vi "LHF.DB.Mongo.Util.VariantToQuery.vi"(0 "Equal":variant, 5 "error in (no error)":errorcluster) -> (14 ".NET Refnum out":refnum<k24>, 19 "error out":errorcluster)   [LabVIEW 2013, in "LHF.DB.Mongo.lvclass"]
uses:
  LHF.DB.Mongo.lvclass
  C:/Users/Ricardo/Desktop/Projetos/LabVIEW-MongoDB/src/Driver/MongoDB.Driver.dll
  LabVIEW-MongoDB/src/Driver/MongoDB.Driver.dll
  C:/Users/Ricardo/Desktop/Projetos/LabVIEW-MongoDB/src/Driver/MongoDB.Bson.dll
  LabVIEW-MongoDB/src/Driver/MongoDB.Bson.dll
  <userlib>/_OpenG.lib/string/string.llb/Trim Whitespace (String)__ogtk.vi
  <vilib>/Utility/VariantDataType/VariantType.lvlib
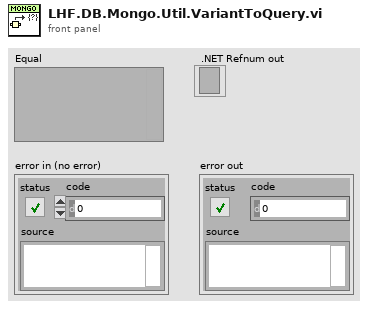
[diagram p1: front panel]
types:
  T1 = typedef "VariantType.lvlib/Type.ctl" = enum8{"Invalid Type", "Void", "I8", "I16", "I32", "I64", "U8", "U16", "U32", "U64", "Single Float", "Double Float", "Extended Float", "Single Complex", "Double Complex", "Extended Complex", "Enum U8", "Enum U16", "Enum U32", "Enum U64", "Single Float With Unit", "Double Float With Unit", "Extended Float With Unit", "Single Complex with Unit", "Double Complex with Unit", "Extended Complex with Unit", "Boolean", "String", "Path", "Picture", "Tag", "Array", "Cluster", "Variant", "LV Variant", "Waveform", "Timestamp", "Digital Waveform", "Digital Data", "ExpressData", "Refnum", "External Data", "VI", "Poly VI", "LabVIEW Class Instance", "Fixed Point"}
  T2 = enum16{"$eq:", "$ne:", "$lte:", "$lt", "$gte:", "$gt:", "<=", "<", ">=", ">", "!=", "==", "!*", "*"}
  T3 = enum16{"$and:", "$and", "&&", "$or:", "$or", "||"}
  T4 = typedef "LHF.DB.Mongo.lvclass/LHF.DB.Mongo.Typedef.VariantData.ctl" = cluster{"Type Enum":T1, "Name":string, "Variant":variant}
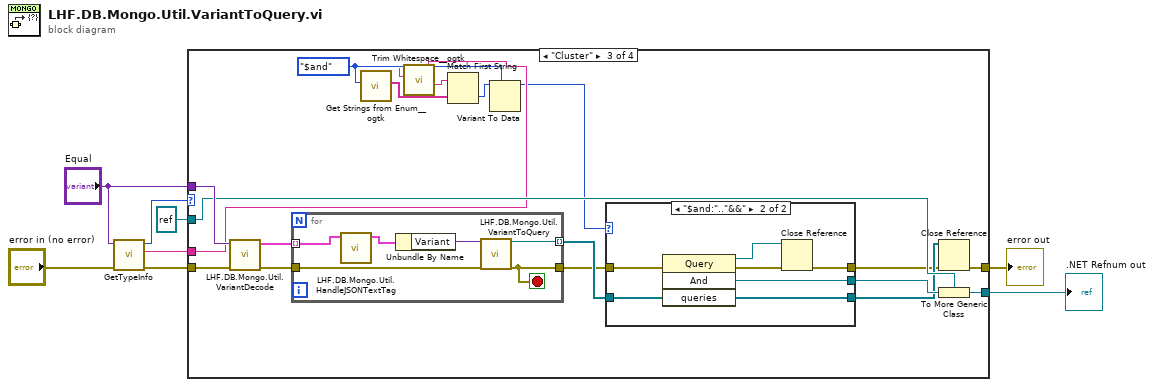
[diagram p0: block diagram]
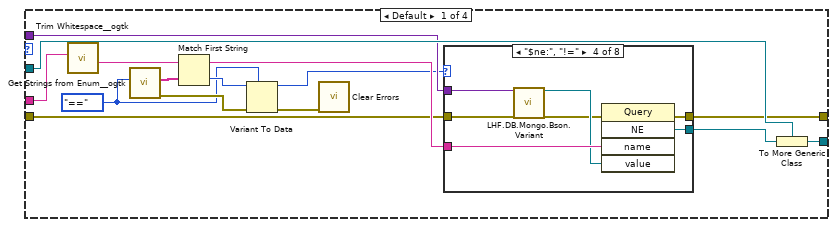
[diagram p2: hidden frame]
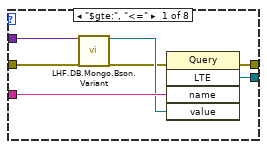
[diagram p3: hidden frame]
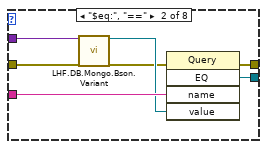
[diagram p4: hidden frame]
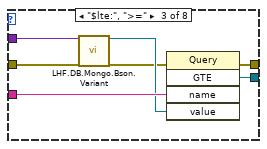
[diagram p5: hidden frame]
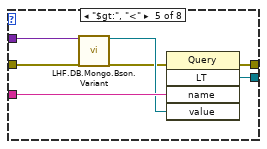
[diagram p6: hidden frame]
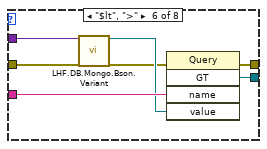
[diagram p7: hidden frame]
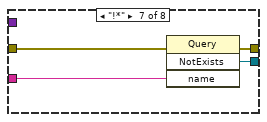
[diagram p8: hidden frame]
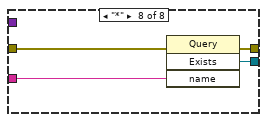
[diagram p9: hidden frame]
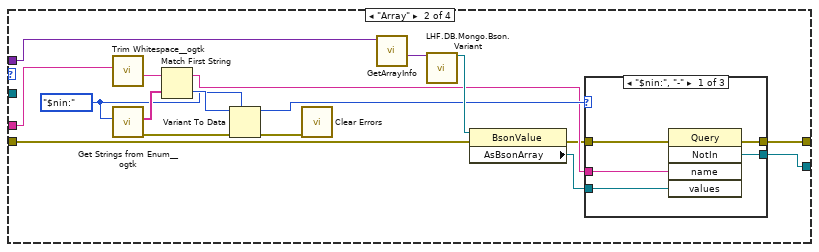
[diagram p10: hidden frame]
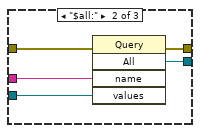
[diagram p11: hidden frame]
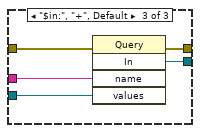
[diagram p12: hidden frame]
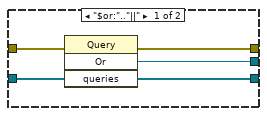
[diagram p13: hidden frame]
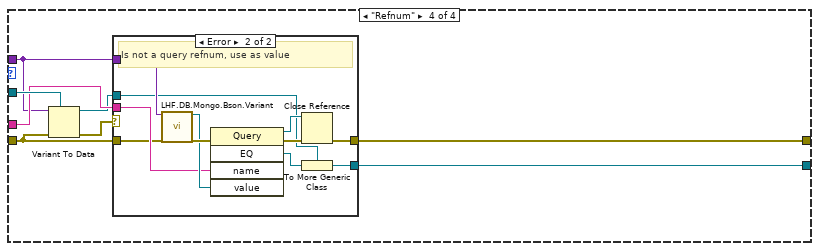
[diagram p14: hidden frame]
diagram:
  n1 = call <vilib>:"GetTypeInfo.vi"("error in (no error)"="error in (no error)", "Variant"="Equal") -> ("error out"=w8:errorcluster, "Name"=w6:string, "Type Enum"=w2:T1)  [unwired: 5 in, 2 out]
  n2 = case shown="\"Cluster\"" w2 {
    tunnel: "Equal" -> [w15 w90 w123 w146]
    tunnel: [w22 w81 w117 w144] -> w4
    tunnel: [w13 w76 w113 w143] -> w5
    tunnel: refnum<k24> refnum ("query") -> [w23 _ w118 w149]
    tunnel: w6 -> [w16 w79 w107 w147]
    tunnel: w8 -> [w12 w74 w112 w142]
    frame Default {
      w10 = T2."=="
      n3 = call-poly <userlib>:"Trim Whitespace__ogtk.vi"("String in"=w16) -> ("String out"=w21:string)  [unwired: 6 in]
      n4 = call <userlib>:"Get Strings from Enum__ogtk.vi"("Enum"=w10) -> ("error out"=w17:errorcluster, "Enum Strings"=w19:string[])  [unwired: 7 in, 2 out]
      n5 = Match First String(2:w19, 3:w21) -> (0:w11:i32, 1:w20:string)
      n6 = Variant To Data(error in=w17, type=w10, Variant=w11) -> (data=w9:T2, error out=w18:errorcluster)
      n7 = call <vilib>:"Clear Errors.vi"("error in (no error)"=w18) -> ()  [unwired: 6 in, 1 out]
      n8 = case shown="\"$ne:\", \"!=\"" w9 {
        tunnel: w15 -> [w27 w35 w42 w50 w56 w63 _ _]
        tunnel: w20 -> [w30 w37 w44 w51 w58 w65 w69 w71]
        tunnel: [w29 w36 w43 w46 w57 w64 w68 w73] -> w14
        tunnel: w12 -> [w24 w33 w39 w48 w54 w61 w66 w70]
        tunnel: [w28 w31 w38 w45 w52 w59 w67 w72] -> w13
        frame "$gte:", "<=" {
          n9 = call "LHF.DB.Mongo.Bson.Variant.vi"("Variant"=w27, "error IO"=w24) -> ("BsonValue"=w26:refnum<k24>, "error IO 2"=w25:errorcluster)  [unwired: 16 in]
          n10 = invoke class="Query" method="LTE"(error in=w25, "name"=w30, "value"=w26) -> (error out=w28:errorcluster, "LTE"=w29:refnum<k24>)  [unwired: 2 in, 3 out]
        }
        frame "$eq:", "==" {
          n11 = call "LHF.DB.Mongo.Bson.Variant.vi"("Variant"=w35, "error IO"=w33) -> ("BsonValue"=w34:refnum<k24>, "error IO 2"=w32:errorcluster)  [unwired: 16 in]
          n12 = invoke class="Query" method="EQ"(error in=w32, "name"=w37, "value"=w34) -> (error out=w31:errorcluster, "EQ"=w36:refnum<k24>)  [unwired: 2 in, 3 out]
        }
        frame "$lte:", ">=" {
          n13 = call "LHF.DB.Mongo.Bson.Variant.vi"("Variant"=w42, "error IO"=w39) -> ("BsonValue"=w41:refnum<k24>, "error IO 2"=w40:errorcluster)  [unwired: 16 in]
          n14 = invoke class="Query" method="GTE"(error in=w40, "name"=w44, "value"=w41) -> (error out=w38:errorcluster, "GTE"=w43:refnum<k24>)  [unwired: 2 in, 3 out]
        }
        frame "$ne:", "!=" {
          n15 = call "LHF.DB.Mongo.Bson.Variant.vi"("Variant"=w50, "error IO"=w48) -> ("BsonValue"=w49:refnum<k24>, "error IO 2"=w47:errorcluster)  [unwired: 16 in]
          n16 = invoke class="Query" method="NE"(error in=w47, "name"=w51, "value"=w49) -> (error out=w45:errorcluster, "NE"=w46:refnum<k24>)  [unwired: 2 in, 3 out]
        }
        frame "$gt:", "<" {
          n17 = call "LHF.DB.Mongo.Bson.Variant.vi"("Variant"=w56, "error IO"=w54) -> ("BsonValue"=w55:refnum<k24>, "error IO 2"=w53:errorcluster)  [unwired: 16 in]
          n18 = invoke class="Query" method="LT"(error in=w53, "name"=w58, "value"=w55) -> (error out=w52:errorcluster, "LT"=w57:refnum<k24>)  [unwired: 2 in, 3 out]
        }
        frame "$lt", ">" {
          n19 = call "LHF.DB.Mongo.Bson.Variant.vi"("Variant"=w63, "error IO"=w61) -> ("BsonValue"=w62:refnum<k24>, "error IO 2"=w60:errorcluster)  [unwired: 16 in]
          n20 = invoke class="Query" method="GT"(error in=w60, "name"=w65, "value"=w62) -> (error out=w59:errorcluster, "GT"=w64:refnum<k24>)  [unwired: 2 in, 3 out]
        }
        frame "!*" {
          n21 = invoke class="Query" method="NotExists"(error in=w66, "name"=w69) -> (error out=w67:errorcluster, "NotExists"=w68:refnum<k24>)  [unwired: 2 in, 2 out]
        }
        frame "*" {
          n22 = invoke class="Query" method="Exists"(error in=w70, "name"=w71) -> (error out=w72:errorcluster, "Exists"=w73:refnum<k24>)  [unwired: 2 in, 2 out]
        }
      }
      n23 = To More Generic Class(target class=w23, reference=w14) -> (generic class reference=w22:refnum<k24>)
    }
    frame "Array" {
      w83 = enum16{"$in:", "$nin:", "$all:", "+", "-"}."$nin:"
      n24 = call-poly <userlib>:"Trim Whitespace__ogtk.vi"("String in"=w79) -> ("String out"=w78:string)  [unwired: 6 in]
      n25 = call <userlib>:"Get Strings from Enum__ogtk.vi"("Enum"=w83) -> ("error out"=w85:errorcluster, "Enum Strings"=w87:string[])  [unwired: 7 in, 2 out]
      n26 = Match First String(2:w87, 3:w78) -> (0:w84:i32, 1:w77:string)
      n27 = Variant To Data(error in=w85, type=w83, Variant=w84) -> (data=w80:enum16{"$in:", "$nin:", "$all:", "+", "-"}, error out=w86:errorcluster)
      n28 = call <vilib>:"Clear Errors.vi"("error in (no error)"=w86) -> ()  [unwired: 6 in, 1 out]
      n29 = call <vilib>:"GetArrayInfo.vi"("Variant"=w90) -> ("ArrayElement"=w89:variant)  [unwired: 7 in, 3 out]
      n30 = call "LHF.DB.Mongo.Bson.Variant.vi"("Variant"=w89) -> ("BsonValue"=w88:refnum<k24>)  [unwired: 17 in, 1 out]
      n31 = property class="BsonValue"(reference=w88, error in=w74) -> (error out=w75:errorcluster, "AsBsonArray"=w82:refnum<k24>)  [unwired: 1 out]
      n32 = case shown="\"$nin:\", \"-\"" w80 {
        tunnel: w77 -> [w95 w100 w105]
        tunnel: w82 -> [w92 w96 w104]
        tunnel: [w94 w99 w103] -> w81
        tunnel: [w93 w98 w102] -> w76
        tunnel: w75 -> [w91 w97 w101]
        frame "$nin:", "-" {
          n33 = invoke class="Query" method="NotIn"(error in=w91, "name"=w95, "values"=w92) -> (error out=w93:errorcluster, "NotIn"=w94:refnum<k24>)  [unwired: 2 in, 3 out]
        }
        frame "$all:" {
          n34 = invoke class="Query" method="All"(error in=w97, "name"=w100, "values"=w96) -> (error out=w98:errorcluster, "All"=w99:refnum<k24>)  [unwired: 2 in, 3 out]
        }
        frame "$in:", "+", Default {
          n35 = invoke class="Query" method="In"(error in=w101, "name"=w105, "values"=w104) -> (error out=w102:errorcluster, "In"=w103:refnum<k24>)  [unwired: 2 in, 3 out]
        }
      }
    }
    frame "Cluster" {
      w109 = T3."$and"
      n36 = call "LHF.DB.Mongo.Util.VariantDecode.vi"("error in (no error)"=w112, "variant"=w123) -> ("error out"=w121:errorcluster, "Variant Data"=w122:T4[])  [unwired: 7 in, 1 out]
      n37 = for {
        tunnel: w122 -> [w141] mode=indexing
        tunnel: [w137] -> w120 mode=indexing
        tunnel: w121 -> [w139]
        tunnel: [w138] -> w116
        stop <- w138 stop-if-true
        n38 = call "LHF.DB.Mongo.Util.HandleJSONTextTag.vi"("Variant Data"=w141) -> ("Variant Data (tag stripped)"=w140:T4)  [unwired: 9 in, 1 out]
        n39 = Unbundle By Name(w140) -> ("Variant"=w136:variant)
        n40 = call "LHF.DB.Mongo.Util.VariantToQuery.vi"("Equal"=w136, "error in (no error)"=w139) -> (".NET Refnum out"=w137:refnum<k24>, "error out"=w138:errorcluster)  [unwired: 16 in]
      }
      n41 = call <userlib>:"Get Strings from Enum__ogtk.vi"("Enum"=w109) -> ("Enum Strings"=w111:string[])  [unwired: 7 in, 3 out]
      n42 = call-poly <userlib>:"Trim Whitespace__ogtk.vi"("String in"=w107) -> ("String out"=w108:string)  [unwired: 6 in]
      n43 = Match First String(2:w111, 3:w108) -> (0:w110:i32)  [unwired: 1 out]
      n44 = Variant To Data(type=w109, Variant=w110) -> (data=w106:T3)  [unwired: 1 in, 1 out]
      n45 = case shown="\"$and:\"..\"&&\"" w106 {
        tunnel: w120 -> [w128 w135]
        tunnel: [w127 w134] -> w119
        tunnel: [w126 w130] -> w114
        tunnel: w116 -> [w125 w133]
        tunnel: [w124 w132] -> w115
        frame "$or:".."||" {
          n46 = invoke class="Query" method="Or"(error in=w125, "queries"=w128) -> (error out=w126:errorcluster, "Or"=w127:refnum<k24>, "queries"=w124:refnum<k24>[])  [unwired: 2 in, 1 out]
        }
        frame "$and:".."&&" {
          n47 = invoke class="Query" method="And"(error in=w133, "queries"=w135) -> (reference out=w129:refnum<k24>, error out=w131:errorcluster, "And"=w134:refnum<k24>, "queries"=w132:refnum<k24>[])  [unwired: 2 in]
          n48 = Close Reference(reference=w129, error in (no error)=w131) -> (error out=w130:errorcluster)
        }
      }
      n49 = Close Reference(reference=w115, error in (no error)=w114) -> (error out=w113:errorcluster)
      n50 = To More Generic Class(target class=w118, reference=w119) -> (generic class reference=w117:refnum<k24>)
    }
    frame "Refnum" {
      n51 = Variant To Data(error in=w142, type=w149, Variant=w146) -> (data=w145:refnum<k24>, error out=w148:errorcluster)
      n52 = case shown="Error" w148 {
        selector: w148 -> [w150 _]
        tunnel: w147 -> [_ w157]
        tunnel: w146 -> [_ w156]
        tunnel: w145 -> [w151 w155]
        tunnel: [w151 w154] -> w144
        tunnel: [w150 w153] -> w143
        tunnel: w142 -> [_ w152]
        frame No Error {
          # "is a query refnum, use it"
        }
        frame Error {
          # "Is not a query refnum, use as value"
          n53 = call "LHF.DB.Mongo.Bson.Variant.vi"("Variant"=w156, "error IO"=w152) -> ("BsonValue"=w158:refnum<k24>, "error IO 2"=w161:errorcluster)  [unwired: 16 in]
          n54 = invoke class="Query" method="EQ"(error in=w161, "name"=w157, "value"=w158) -> (reference out=w162:refnum<k24>, error out=w160:errorcluster, "EQ"=w159:refnum<k24>)  [unwired: 2 in, 2 out]
          n55 = Close Reference(reference=w162, error in (no error)=w160) -> (error out=w153:errorcluster)
          n56 = To More Generic Class(target class=w155, reference=w159) -> (generic class reference=w154:refnum<k24>)
        }
      }
    }
  }
  "error out" <- w5
  ".NET Refnum out" <- w4
